vi "Merch Process Weekly.vi"() -> ()   [LabVIEW 2010]
uses:
  <vilib>/regexp/Match Regular Expression.xnode
panel:
  out "Current File Number":i32
  out "Compare 2":string
  out "Compare 1":string
  out "Numeric":i32
  out "Most Recent File Path":path
  out "date":string
  out "appended path":path
  out "File Name":string
  out "filenames":string[](array[string])
  out "Number of Files":i32
  out "name":string
  out "Resulting Time Stamp":timestamp
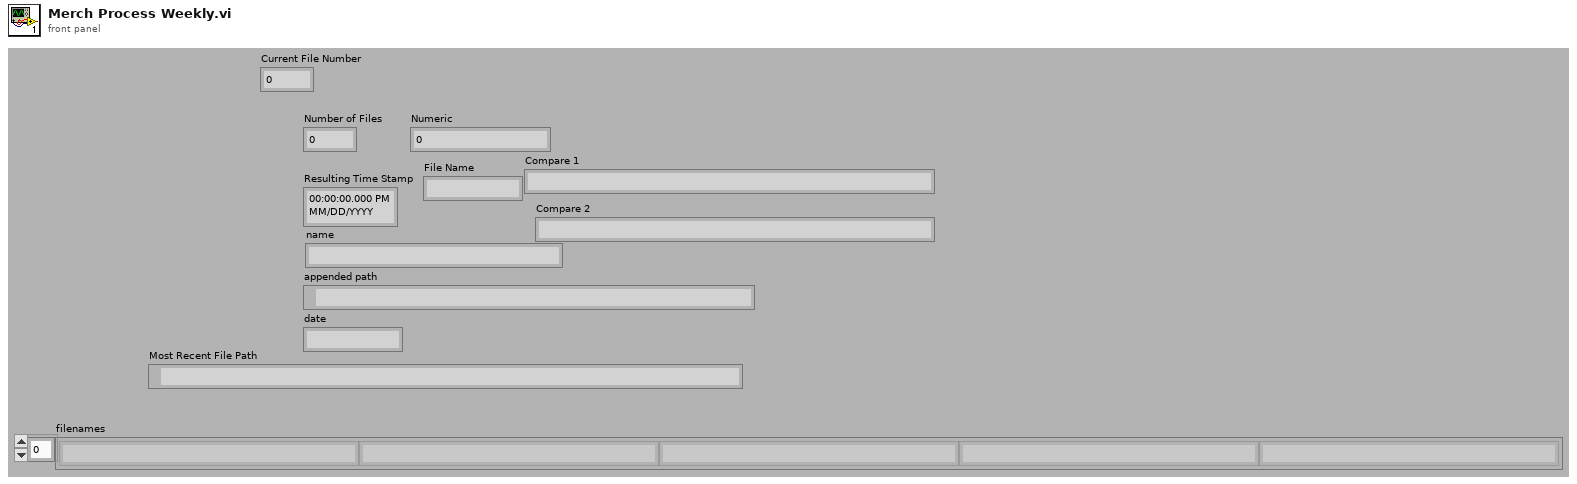
[diagram p1: front panel]
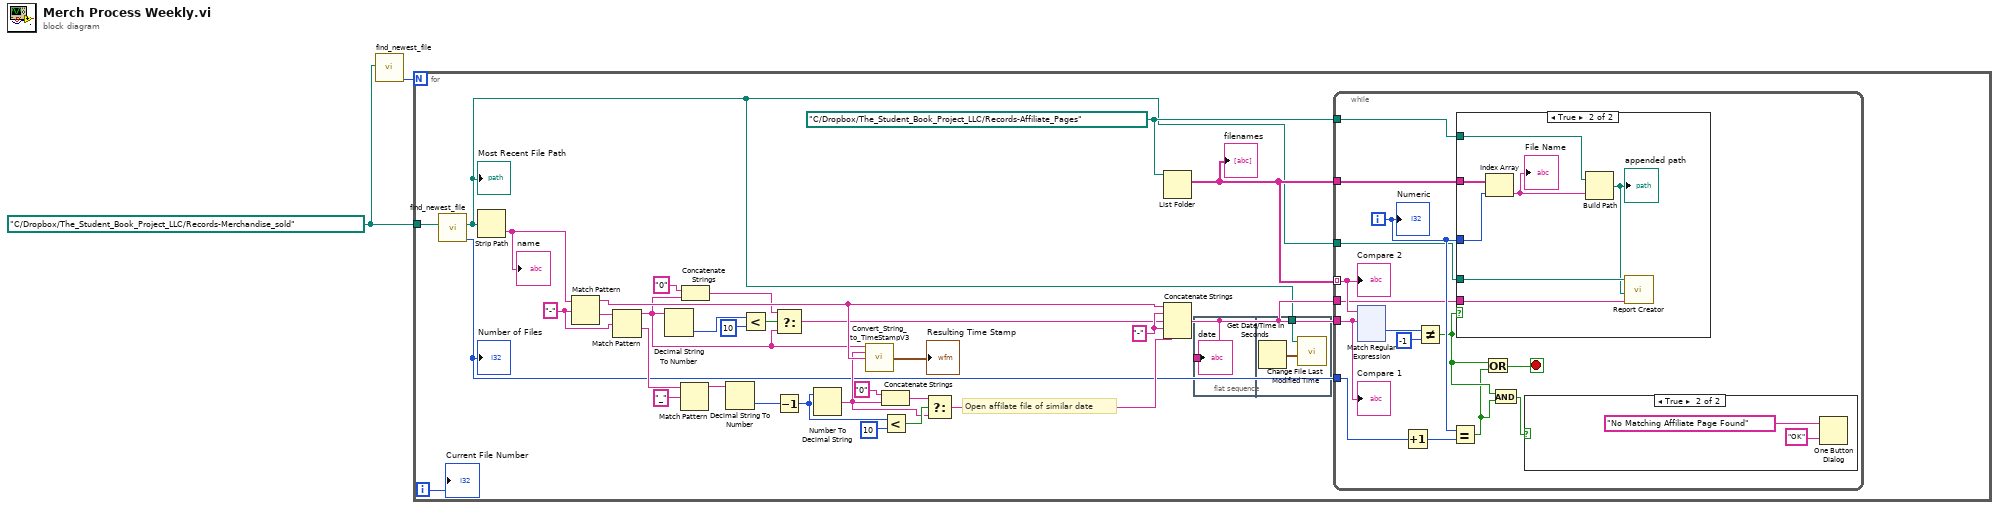
[diagram p0: block diagram]
diagram:
  w1 = path "C:/Dropbox/The_Student_Book_Project_LLC/Records-Merchandise_sold" ("Directory Path to Start the Search")
  n1 = call "find_newest_file.vi"("Directory Path to Start the Search"=w1) -> ("Number of Files"=w2:i32)  [unwired: 9 in, 1 out]
  n2 = for {
    N: w2 -> [_]
    tunnel: w1 -> [w5]
    i -> [w3]
    w26 = "-" ("string")
    w24 = path "C:/Dropbox/The_Student_Book_Project_LLC/Records-Affiliate_Pages" ("Directory Path to Start the Search")
    w31 = "-" ("regular expression")
    # "Open affilate file of similar date"
    n3 = call "find_newest_file.vi"("Directory Path to Start the Search"=w5) -> ("Number of Files"=w6:i32, "Most Recent File Path"=w4:path)  [unwired: 9 in]
    "Number of Files" <- w6
    "Most Recent File Path" <- w4
    n4 = Strip Path(path=w4) -> (name=w33:string)  [unwired: 1 out]
    "name" <- w33
    n5 = Match Pattern(string=w33, regular expression=w31) -> (before substring=w27:string, after substring=w32:string)  [unwired: 1 in, 2 out]
    n6 = Match Pattern(string=w32, regular expression=w31) -> (before substring=w8:string, after substring=w30:string)  [unwired: 1 in, 2 out]
    n7 = Decimal String To Number(string=w8) -> (number=w10:i32)  [unwired: 2 in, 1 out]
    n8 = Match Pattern(string=w30, regular expression="_") -> (before substring=w21:string)  [unwired: 1 in, 3 out]
    n9 = Concatenate Strings("0" ("string"), w8) -> (w11:string)
    n10 = Decimal String To Number(string=w21) -> (number=w22:i32)  [unwired: 2 in, 1 out]
    n11 = Less?(x=w10, y=10) -> (x < y?=w12:bool)
    n12 = Select(t=w11, s=w12, f=w8) -> (s? t:f=w7:string)
    n13 = Decrement(x=w22) -> (x-1=w20:i32)
    n14 = Number To Decimal String(number=w20) -> (decimal integer string=w15:string)  [unwired: 1 in]
    n15 = call "Convert_String_to_TimeStampV3.vi"("Month (number)"=w8, "day"=w15, "Year"=w27) -> ("Resulting Time Stamp"=→"Resulting Time Stamp":timestamp)  [unwired: 12 in]
    n16 = Concatenate Strings("0" ("string"), w15) -> (w16:string)
    n17 = Less?(x=w20, y=10) -> (x < y?=w17:bool)
    n18 = Select(t=w16, s=w17, f=w15) -> (s? t:f=w14:string)
    n19 = List Folder(path=w24) -> (filenames=w25:string[])  [unwired: 3 in, 3 out]
    "filenames" <- w25
    n20 = Concatenate Strings(w27, w26, w7, w26, w14) -> (w23:string)
    n21 = flat-sequence {
      tunnel: w23 -> [w34]
      tunnel: w4 -> [w35]
      frame #0 {
        "date" <- w34
      }
      frame #1 {
        n22 = Get Date/Time In Seconds() -> (seconds since 1Jan1904=w36:timestamp)
        n23 = call "Change File Last Modified Time.vi"("lastWriteTime"=w36, "File path"=w35) -> ()  [unwired: 9 in, 1 out]
      }
    }
    n24 = while {
      tunnel: w25 -> [w51] mode=indexing
      tunnel: w25 -> [w48]
      tunnel: w24 -> [w47]
      tunnel: w23 -> [w46]
      tunnel: w6 -> [w44]
      tunnel: w4 -> [w42]
      tunnel: w23 -> [w41]
      i -> [w45]
      stop <- w40 stop-if-true
      n25 = xnode "Match Regular Expression"("input string"=w51, "regular expression"=w46) -> ("offset past match"=w50:i32)  [unwired: 4 in, 4 out]
      n26 = Increment(x=w44) -> (x+1=w43:i32)
      n27 = Not Equal?(x=w50, y=-1) -> (x != y?=w39:bool)
      n28 = Equal?(x=w45, y=w43) -> (x = y?=w38:bool)
      n29 = case shown="True" w39 {
        tunnel: w48 -> [_ w60]
        tunnel: w45 -> [_ w59]
        tunnel: w47 -> [_ w58]
        tunnel: w42 -> [_ w56]
        tunnel: w41 -> [_ w55]
        frame False {
        }
        frame True {
          n30 = Index Array(array=w60, index=w59) -> (element=w57:string)
          "File Name" <- w57
          n31 = Build Path(base path=w58, name or relative path=w57) -> (appended path=w54:path)
          "appended path" <- w54
          n32 = call "Report Creator.vi"("date"=w55, "Affiliate Weekly Path"=w54, "Merch Weekly Path"=w56) -> ()  [unwired: 9 in]
        }
      }
      n33 = Or(x=w39, y=w38) -> (x .or. y?=w40:bool)
      n34 = And(x=w39, y=w38) -> (x .and. y?=w37:bool)
      n35 = case shown="True" w37 {
        frame False {
        }
        frame True {
          n36 = One Button Dialog(message="No Matching Affiliate Page Found", button name ("OK")="OK") -> ()  [unwired: 1 out]
        }
      }
      "Numeric" <- w45
      "Compare 1" <- w46
      "Compare 2" <- w51
    }
    "Current File Number" <- w3
  }
